vi "DoMeasureSamples.vi"(8 "Error In":errorcluster, 10 "TLCamera reference in":refnum<k24>, 11 "MotorController in":refnum<class "MotorController.lvclass">) -> (0 "Error Out":errorcluster, 2 "TLCamera reference out":refnum<k24>, 3 "MotorController out":refnum<class "MotorController.lvclass">)   [LabVIEW 2019]
uses:
  C:/Users/jleeman/git_repos/CAxis_Machine/C-Axis LabView Controller/Library_X64/Thorlabs.TSI.TLCameraInterfaces.dll
  Library_X64/Thorlabs.TSI.TLCameraInterfaces.dll
  MotorController.lvclass
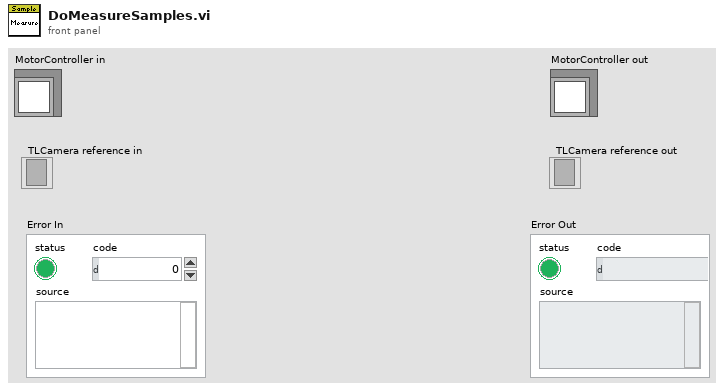
[diagram p1: front panel]
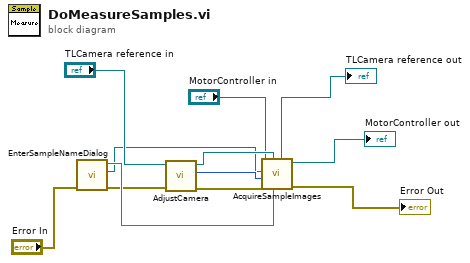
[diagram p0: block diagram]
diagram:
  n1 = call "EnterSampleNameDialog.vi"("Error In"="Error In") -> ("Error Out"=w3:errorcluster, "Schedule File out"=w1:path, "Sample Name"=w12:string)  [unwired: 8 in]
  n2 = call "AdjustCamera.vi"("Error In"=w3, "TLCamera reference in"="TLCamera reference in") -> ("Error Out"=w2:errorcluster, "Exposure (us)"=w11:u32, "TLCamera reference out"=w9:refnum<k24>)  [unwired: 7 in]
  n3 = call "AcquireSampleImages.vi"("SampleName"=w12, "TLCamera reference in"=w9, "Error In"=w2, "Exposure"=w11, "Schedule File"=w1, "MotorController in"="MotorController in") -> ("Error Out"=→"Error Out":errorcluster, "MotorController out"=→"MotorController out":refnum<class "MotorController.lvclass">, "TLCamera reference out"=→"TLCamera reference out":refnum<k24>)  [unwired: 3 in]
